vi "Ramp delta.vi"(9 "start":dbl, 10 "delta":dbl, 11 "samples":i32) -> (2 "last value":dbl, 3 "ramp signal":dbl[](array[numeric]))   [LabVIEW 2013]
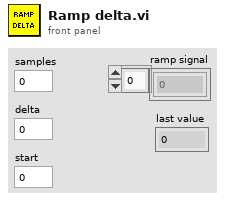
[diagram p1: front panel]
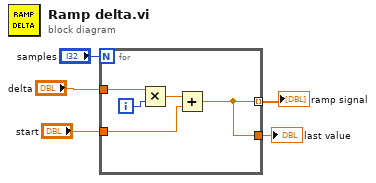
[diagram p0: block diagram]
diagram:
  n1 = for {
    N: "samples" -> [_]
    tunnel: "start" -> [w7]
    tunnel: "delta" -> [w9]
    tunnel: [w6] -> w2 mode=indexing
    tunnel: [w6] -> w1
    i -> [w10]
    n2 = Multiply(x=w9, y=w10) -> (x*y=w8:dbl)
    n3 = Add(x=w8, y=w7) -> (x+y=w6:dbl)
  }
  "ramp signal" <- w2
  "last value" <- w1
